vi "SJ_3D_Surfacer.vi"(1 "SJ Array Input":dbl[](array[numeric])) -> (0 "3D Plot out":refnum<class "3D Plot Datatype.lvclass">[](array[class]))   [LabVIEW 2011]
uses:
  <vilib>/Math Plots/3D Math Plots/3D Plot/3D Plot Datatype/3D Plot Datatype.lvclass
  Acquisition/Data_Translation/DataTranslation_global.vi
  <vilib>/Math Plots/3D Math Plots/3D Surface/3D Surface Datatype/Public/Plot Helper (Vector).vi
  <vilib>/Math Plots/3D Math Plots/3D Surface/3D Surface Datatype/3D Surface Datatype.lvclass
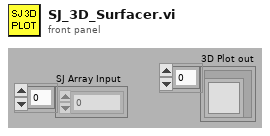
[diagram p1: front panel]
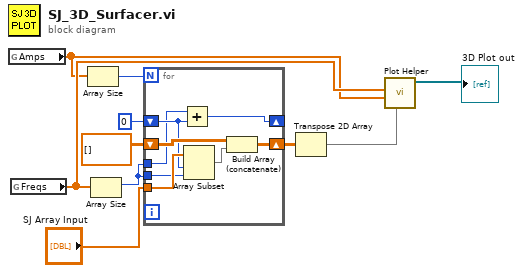
[diagram p0: block diagram]
diagram:
  n1 = global read "DataTranslation_global.vi" "Amps"() -> (w2:dbl[])
  n2 = global read "DataTranslation_global.vi" "Freqs"() -> (w3:dbl[])
  n3 = Array Size(array=w2) -> (size(s)=w6:i32)
  n4 = Array Size(array=w3) -> (size(s)=w5:i32)
  n5 = for {
    N: w6 -> [_]
    tunnel: "SJ Array Input" -> [w15]
    shift-right: [w18] -> _
    shift-left: 0 -> [w14]
    shift-right: [w17] -> w8
    shift-left: dbl[][] [] -> [w16]
    tunnel: w5 -> [w13]
    tunnel: w5 -> [w11]
    n6 = Add(x=w11, y=w14) -> (x+y=w18:i32)
    n7 = Array Subset(array=w15, index=w14, length=w13) -> (w12:dbl[])
    n8 = Build Array (concatenate)(w16, w12) -> (w17:dbl[][])
  }
  n9 = Transpose 2D Array(2D array=w8) -> (transposed array=w4:dbl[][])
  n10 = call-poly <vilib>:"Plot Helper.vi"("z matrix"=w4, "y vector"=w2, "x vector"=w3) -> ("3D Plot lvclass Array out"=→"3D Plot out":refnum<class "3D Plot Datatype.lvclass">[])  [unwired: 3 in, 5 out]
